vi "Test Get Lifecycle Uninitialized.vi"(8 "error in (no error)":errorcluster, 11 "Debug State Analyzer Test In":refnum<class "Debug State Analyzer Test.lvclass">) -> (0 "error out":errorcluster, 3 "Debug State Analyzer Test Out":refnum<class "Debug State Analyzer Test.lvclass">)   [LabVIEW 2020, in "Debug State Analyzer Test.lvclass"]
uses:
  Debug State Analyzer Test.lvclass
  Debug State Analyzer Test.lvclass/Debug State Analyzer Test.ctl
  01074fa8-ee8a-411d-bc8b-fc92c4f90959.vi
  source/State Analyzer/Debug State Analyzer.lvclass
  source/Debug Data/Raw Debug Data.ctl
  source/Debug Data/Debug Data.lvclass
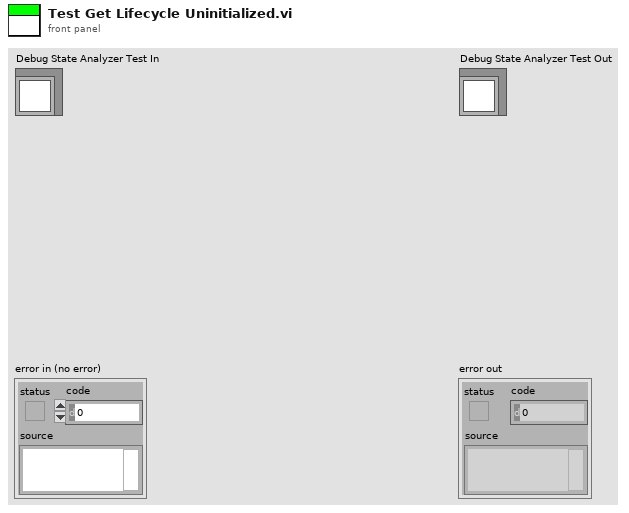
[diagram p1: front panel]
types:
  T1 = typedef "Debug Data.lvclass/Raw Debug Data.ctl" = cluster{"Action":string, "Call Chain":string, "Process":string, "Message":string, "Message Data":variant, "Time":dbl}
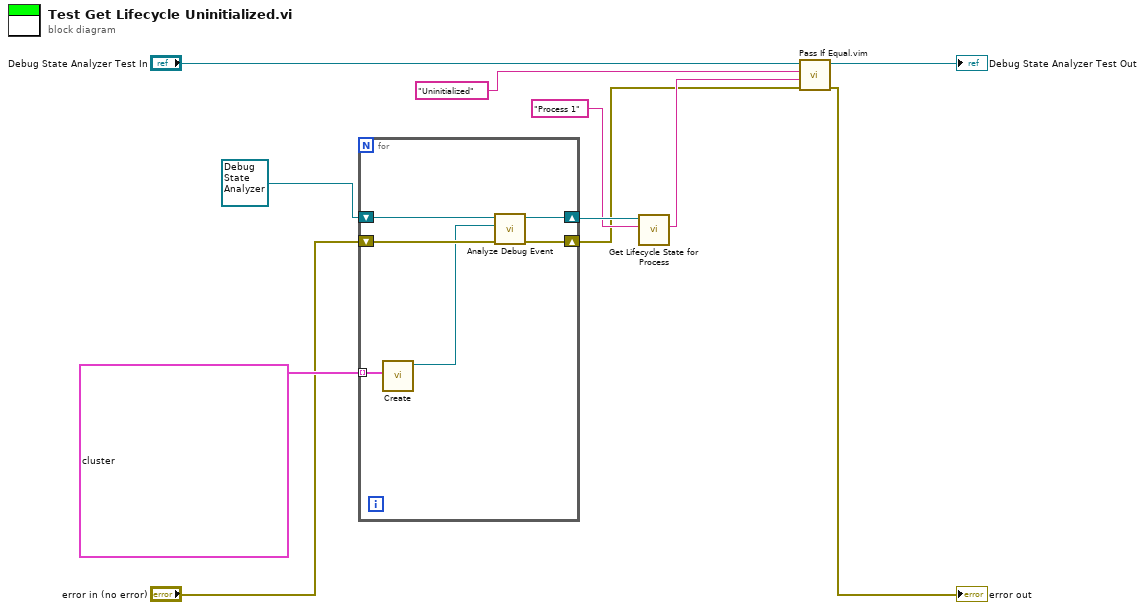
[diagram p0: block diagram]
diagram:
  n1 = for {
    tunnel: T1[] [{"Action"="Send", "Call Chain"="Test.vi:123456", "Process"="Process 1", "Message"="Init", "Message Data"=variant, "Time"=0.0}] ("Debug Data Cluster") -> [w17] mode=indexing
    shift-right: [w15] -> w4
    shift-left: refnum<class "Debug State Analyzer.lvclass"> refnum ("Debug State Analyzer in") -> [w16]
    shift-right: [w13] -> w1
    shift-left: "error in (no error)" -> [w14]
    n2 = call "Create.vi"("Debug Data Cluster"=w17) -> ("Debug Data out"=w12:refnum<class "Debug Data.lvclass">)  [unwired: 9 in, 1 out]
    n3 = call "Analyze Debug Event.vi"("error in (no error)"=w14, "Debug Data.lvclass"=w12, "Debug State Analyzer In"=w16) -> ("error out"=w13:errorcluster, "Debug State Analyzer Out"=w15:refnum<class "Debug State Analyzer.lvclass">)  [unwired: 7 in]
  }
  n4 = call "Get Lifecycle State for Process.vi"("Process"="Process 1", "Debug State Analyzer In"=w4) -> ("Lifecycle State"=w2:string)  [unwired: 8 in, 1 out]
  n5 = call "Pass If Equal.vim"("error in (no error)"=w1, "Actual"=w2, "Expected"="Uninitialized", "LUnit Test Case In"="Debug State Analyzer Test In") -> ("error out"=→"error out":errorcluster, "LUnit Test Case Out"=→"Debug State Analyzer Test Out":refnum<class "Debug State Analyzer Test.lvclass">)  [unwired: 6 in]
